vi "LVClass_Camera get all camera parameter values.vi"(0 "Camera in":refnum<class "Camera.lvclass">, 11 "error in (no error)":errorcluster) -> (4 "Camera out":refnum<class "Camera.lvclass">, 6 "ListOfSettableAndGettableValue":T1[](array[typedef]), 8 "nb_image":u32, 10 "BG Image OUT":refnum<class "Image.lvclass">, 15 "error out":errorcluster)   [LabVIEW 2020, in "Camera.lvclass"]
uses:
  Camera.lvclass
  CameraParametersSetup.ctl
  CameraParameters_Type.ctl
  Image.lvclass
  Camera.lvclass/Camera.ctl
  LVClass_Camera_ Read acquisition state.vi
  LVClass_Camera Read all camera parameters.vi
  LVClass_Image read Image Compat ptr.vi
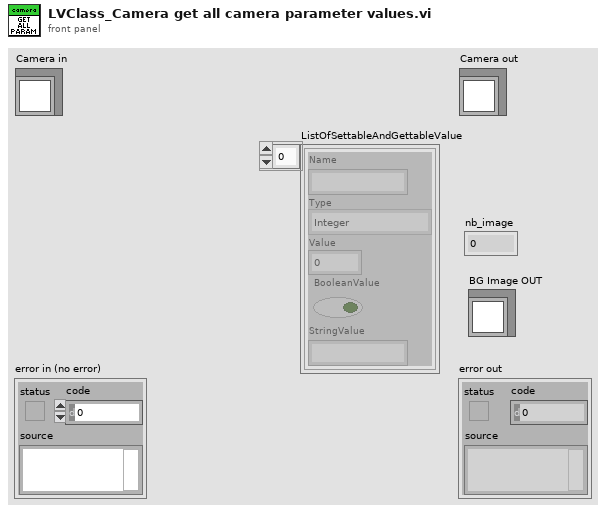
[diagram p1: front panel]
types:
  T1 = typedef "CameraParametersSetup.ctl" = cluster{"Name":string, "Type":T2, "Value":dbl, "BooleanValue":bool, "StringValue":string}
  T2 = typedef "CameraParameters_Type.ctl" = enum16{"Integer", "Real", "String", "Boolean"}
  T3 = typedef "CameraAcquisitionState.ctl" = enum16{"Stop", "Live"}
  T4 = typedef "ParameterID.ctl" = cluster{"Name":string, "Type":T2, "Authorization":T5, "OnFlyAuthorization":T6, "StringDefault":string, "Default":dbl, "Min":dbl, "Max":dbl, "Boolean":bool, "StringParameterList":string[]}
  T5 = typedef "CameraParameters_Authorization.ctl" = enum16{"Disable", "Gettable", "Settable - Gettable"}
  T6 = typedef "CameraParameters_OnFlyAuthorization.ctl" = enum16{"None", "Gettable", "Settable", "Settable - Gettable"}
  T7 = enum32{"invalid app kind", "Development System", "Run Time System", "Student Edition", "Embedded LabVIEW", "Evaluation", "Custom"}
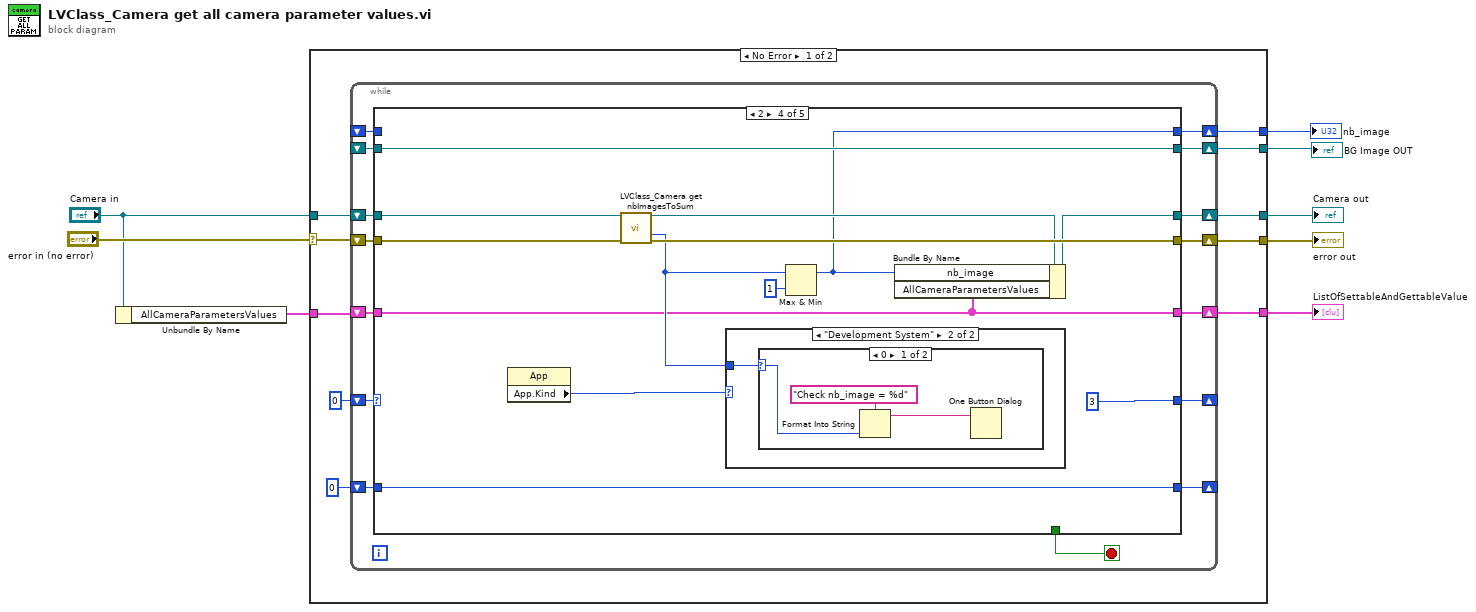
[diagram p0: block diagram]
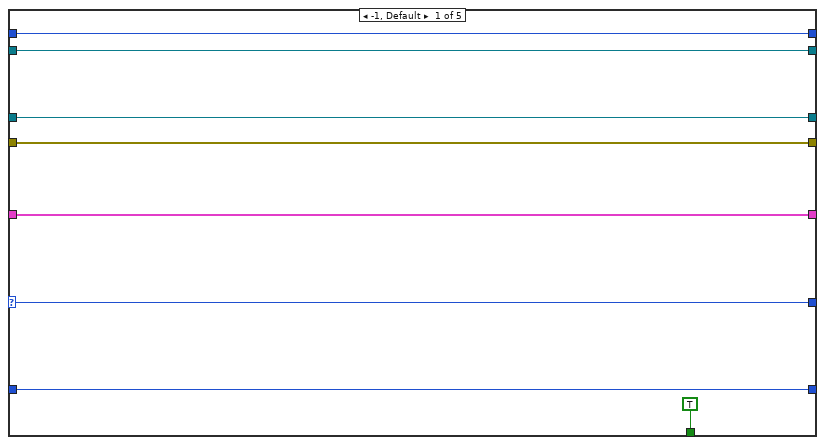
[diagram p2: hidden frame]
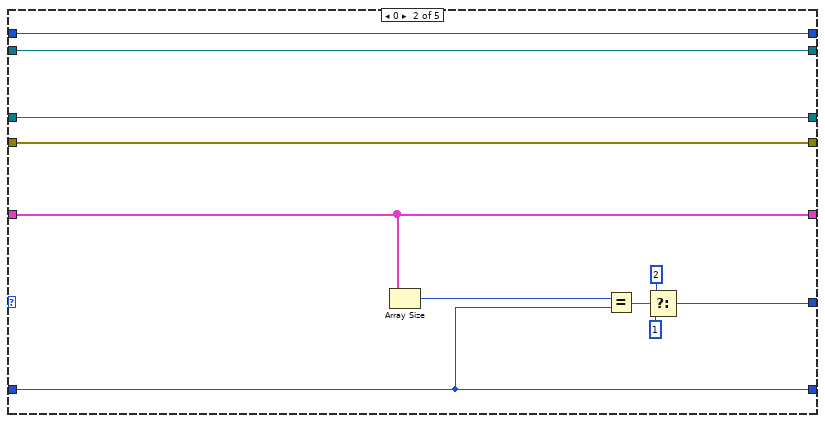
[diagram p3: hidden frame]
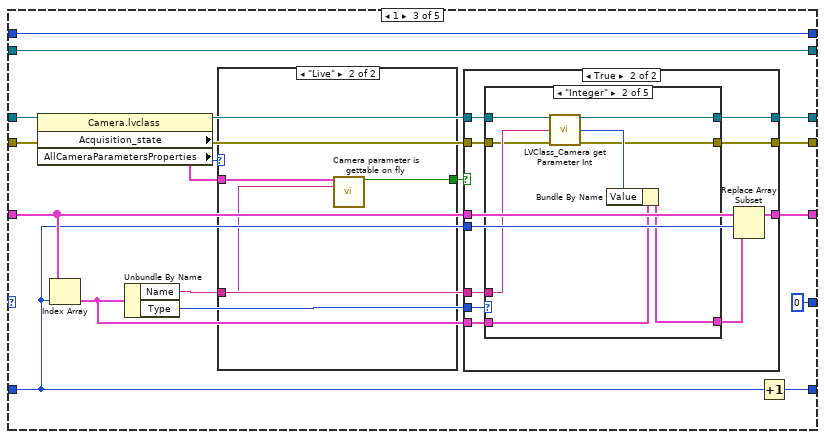
[diagram p4: hidden frame]
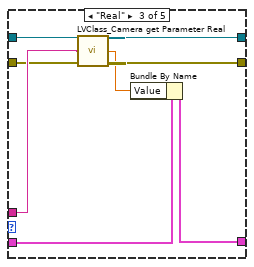
[diagram p7: hidden frame]
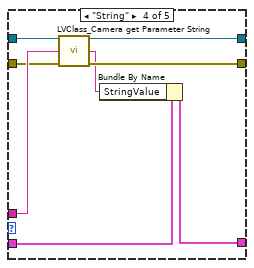
[diagram p8: hidden frame]
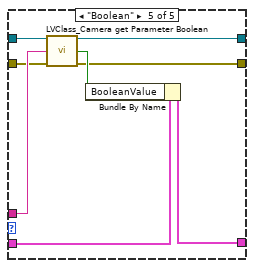
[diagram p9: hidden frame]
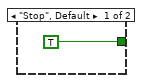
[diagram p10: hidden frame]
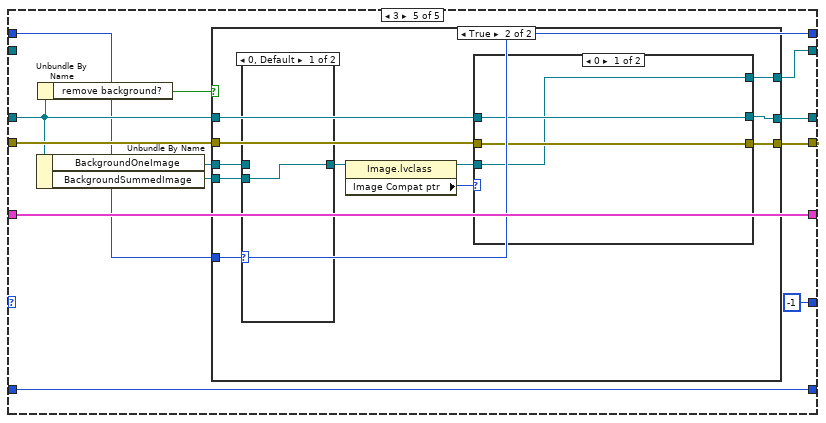
[diagram p13: hidden frame]
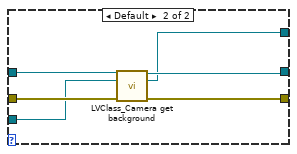
[diagram p16: hidden frame]
diagram:
  n1 = Unbundle By Name("Camera in") -> ("AllCameraParametersValues"=w1:T1[])
  n2 = case shown="No Error" "error in (no error)" {
    selector: "error in (no error)" -> [w14 w180]
    tunnel: [w15 w180] -> w7
    tunnel: [w16 w179] -> w6
    tunnel: "Camera in" -> [w18 w179]
    tunnel: [w13 _] -> w5
    tunnel: [w12 _] -> w4
    tunnel: [w11 _] -> w3
    tunnel: w1 -> [w9 _]
    frame No Error {
      n3 = while {
        shift-right: [w32] -> _
        shift-left: 0 -> [w31]
        shift-right: [w29] -> w15
        shift-left: w14 -> [w28]
        shift-right: [w30] -> w16
        shift-left: w18 -> [w33]
        shift-right: [w25] -> w13
        shift-left: _ -> [w26]
        shift-right: [w24] -> w12
        shift-left: w9 -> [w23]
        shift-right: [w22] -> w11
        shift-left: _ -> [w21]
        shift-right: [w19] -> _
        shift-left: 0 -> [w20]
        stop <- w27 stop-if-true
        n4 = case shown="2" w31 {
          selector: w31 -> [w34 _ _ _ _]
          tunnel: w33 -> [w40 w52 w60 w136 w147]
          tunnel: w28 -> [w39 w51 w58 w135 w153]
          tunnel: [w34 w43 0 3 -1] -> w32
          tunnel: [w40 w52 w70 w131 w152] -> w30
          tunnel: [w39 w51 w69 w134 w151] -> w29
          tunnel: [TRUE _ _ _ _] -> w27
          tunnel: w26 -> [w38 w50 w68 w133 _]
          tunnel: [w38 w50 w68 w133 w150] -> w25
          tunnel: [w36 w48 w62 w125 w149] -> w24
          tunnel: w23 -> [w36 w48 w64 w125 w149]
          tunnel: [w37 w49 w67 w128 w144] -> w22
          tunnel: w21 -> [w37 w49 w67 _ w144]
          tunnel: w20 -> [w35 w46 w63 w130 w142]
          tunnel: [w35 w46 w66 w130 w142] -> w19
          frame -1, Default {
          }
          frame 0 {
            n5 = Array Size(array=w48) -> (size(s)=w47:i32)
            n6 = Equal?(x=w47, y=w46) -> (x = y?=w45:bool)
            n7 = Select(t=2, s=w45, f=1) -> (s? t:f=w43:i32)
          }
          frame 1 {
            n8 = property class="Camera.lvclass"(reference=w60, error in=w58) -> (reference out=w59:refnum<class "Camera.lvclass">, error out=w57:errorcluster, "Acquisition_state"=w56:T3, "AllCameraParametersProperties"=w55:T4[])
            n9 = Index Array(array=w64, index=w63) -> (element=w65:T1)
            n10 = Unbundle By Name(w65) -> ("Name"=w53:string, "Type"=w61:T2)
            n11 = case shown="\"Live\"" w56 {
              tunnel: w55 -> [_ w123]
              tunnel: [TRUE w124] -> w54
              tunnel: w53 -> [_ w122]
              frame "Stop", Default {
              }
              frame "Live" {
                n12 = call "Camera parameter is gettable on fly.vi"("AllCameraParameters"=w123, "Name"=w122) -> ("Gettable?"=w124:bool)  [unwired: 13 in]
              }
            }
            n13 = case shown="True" w54 {
              tunnel: [w74 w85] -> w70
              tunnel: [w73 w84] -> w69
              tunnel: w65 -> [_ w83]
              tunnel: w64 -> [w72 w82]
              tunnel: w63 -> [_ w81]
              tunnel: [w72 w80] -> w62
              tunnel: w61 -> [_ w79]
              tunnel: w53 -> [_ w78]
              tunnel: w59 -> [w74 w77]
              tunnel: w57 -> [w73 w76]
              frame False {
              }
              frame True {
                n14 = case shown="\"Integer\"" w79 {
                  tunnel: w83 -> [w86 w96 w97 w105 w114]
                  tunnel: [w86 w95 w98 w112 w113] -> w75
                  tunnel: w78 -> [_ w94 w103 w109 w119]
                  tunnel: w77 -> [w88 w93 w104 w111 w120]
                  tunnel: [w88 w92 w100 w110 w117] -> w85
                  tunnel: [w87 w90 w101 w107 w115] -> w84
                  tunnel: w76 -> [w87 w89 w102 w108 w118]
                  frame Default {
                  }
                  frame "Integer" {
                    n15 = call "LVClass_Camera get Parameter Int.vi"("Camera in"=w93, "parameter_name"=w94, "error in (no error)"=w89) -> ("Camera out"=w92:refnum<class "Camera.lvclass">, "value"=w91:i32, "error out"=w90:errorcluster)  [unwired: 10 in]
                    n16 = Bundle By Name(cluster=w96, "Value"=w91) -> (w95:T1)
                  }
                  frame "Real" {
                    n17 = call "LVClass_Camera get Parameter Real.vi"("Camera in"=w104, "parameter_name"=w103, "error in (no error)"=w102) -> ("Camera out"=w100:refnum<class "Camera.lvclass">, "value"=w99:dbl, "error out"=w101:errorcluster)  [unwired: 10 in]
                    n18 = Bundle By Name(cluster=w97, "Value"=w99) -> (w98:T1)
                  }
                  frame "String" {
                    n19 = call "LVClass_Camera get Parameter String.vi"("Camera in"=w111, "parameter_name"=w109, "error in (no error)"=w108) -> ("Camera out"=w110:refnum<class "Camera.lvclass">, "value"=w106:string, "error out"=w107:errorcluster)  [unwired: 10 in]
                    n20 = Bundle By Name(cluster=w105, "StringValue"=w106) -> (w112:T1)
                  }
                  frame "Boolean" {
                    n21 = call "LVClass_Camera get Parameter Boolean.vi"("Camera in"=w120, "parameter_name"=w119, "error in (no error)"=w118) -> ("Camera out"=w117:refnum<class "Camera.lvclass">, "value"=w116:bool, "error out"=w115:errorcluster)  [unwired: 10 in]
                    n22 = Bundle By Name(cluster=w114, "BooleanValue"=w116) -> (w113:T1)
                  }
                }
                n23 = Replace Array Subset(array=w82, new element=w75, index=w81) -> (w80:T1[])
              }
            }
            n24 = Increment(x=w63) -> (x+1=w66:i32)
          }
          frame 2 {
            n25 = property class="App"() -> ("App.Kind"=w127:T7)  [unwired: 2 in, 2 out]
            n26 = call "LVClass_Camera get nbImagesToSum.vi"("Camera in"=w136, "error in (no error)"=w135) -> ("Camera out"=w132:refnum<class "Camera.lvclass">, "nb_image"=w126:u32, "error out"=w134:errorcluster)  [unwired: 11 in]
            n27 = case shown="\"Development System\"" w127 {
              tunnel: w126 -> [_ w138]
              frame "invalid app kind", Default {
              }
              frame "Development System" {
                n28 = case shown="0" w138 {
                  selector: w138 -> [w141 _]
                  frame 0 {
                    n29 = Format Into String(format string="Check nb_image = %d" ("message"), w141) -> (resulting string=w139:string)  [unwired: 2 in, 1 out]
                    n30 = One Button Dialog(message=w139) -> ()  [unwired: 1 in, 1 out]
                  }
                  frame 1, Default {
                  }
                }
              }
            }
            n31 = Max & Min(x=w126, y=u32 1) -> (max(x,y)=w128:u32)  [unwired: 1 out]
            n32 = Bundle By Name(cluster=w132, "nb_image"=w128, "AllCameraParametersValues"=w125) -> (w131:refnum<class "Camera.lvclass">)
          }
          frame 3 {
            n33 = Unbundle By Name(w147) -> ("BackgroundOneImage"=w148:refnum<class "Image.lvclass">, "BackgroundSummedImage"=w143:refnum<class "Image.lvclass">)
            n34 = Unbundle By Name(w147) -> ("remove background?"=w145:bool)
            n35 = case shown="True" w145 {
              tunnel: w153 -> [w154 w166]
              tunnel: [w155 w165] -> w152
              tunnel: [w154 w164] -> w151
              tunnel: [w156 w163] -> w150
              tunnel: w148 -> [w156 w159]
              tunnel: w147 -> [w155 w162]
              tunnel: w144 -> [_ w160]
              tunnel: w143 -> [_ w157]
              frame False {
              }
              frame True {
                n36 = case shown="0, Default" w160 {
                  tunnel: w159 -> [_ w169]
                  tunnel: [w168 w169] -> w158
                  tunnel: w157 -> [w168 _]
                  frame 0, Default {
                  }
                  frame 1 {
                  }
                }
                n37 = property class="Image.lvclass"(reference=w158) -> (reference out=w161:refnum<class "Image.lvclass">, "Image Compat ptr"=w167:i32)  [unwired: 1 in, 1 out]
                n38 = case shown="0" w167 {
                  tunnel: w162 -> [w171 w178]
                  tunnel: w166 -> [w172 w177]
                  tunnel: [w171 w176] -> w165
                  tunnel: [w172 w175] -> w164
                  tunnel: [w170 w174] -> w163
                  tunnel: w161 -> [w170 w173]
                  frame 0 {
                  }
                  frame Default {
                    n39 = call "LVClass_Camera get background.vi"("Camera in"=w178, "Image.lvclass"=w173, "error in (no error)"=w177) -> ("Camera out"=w176:refnum<class "Camera.lvclass">, "Image.lvclass"=w174:refnum<class "Image.lvclass">, "error out"=w175:errorcluster)  [unwired: 10 in]
                  }
                }
              }
            }
          }
        }
      }
    }
    frame Error {
    }
  }
  "error out" <- w7
  "Camera out" <- w6
  "ListOfSettableAndGettableValue" <- w4
  "nb_image" <- w3
  "BG Image OUT" <- w5
